vi "set_new_position.vi"(8 "error in (no error)":errorcluster, 10 "set_pos":dbl[](array[numeric]), 11 "dummyStage in":refnum<class "dummyStage.lvclass">) -> (0 "error out":errorcluster, 3 "dummyStage out":refnum<class "dummyStage.lvclass">)   [LabVIEW 2019, in "dummyStage.lvlib" / "dummyStage.lvclass"]
uses:
  dummyStage.lvclass
  subVIs/stage_idling.vi
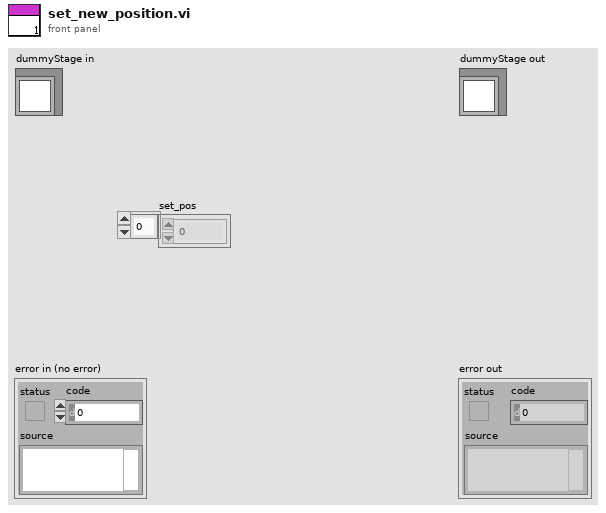
[diagram p1: front panel]
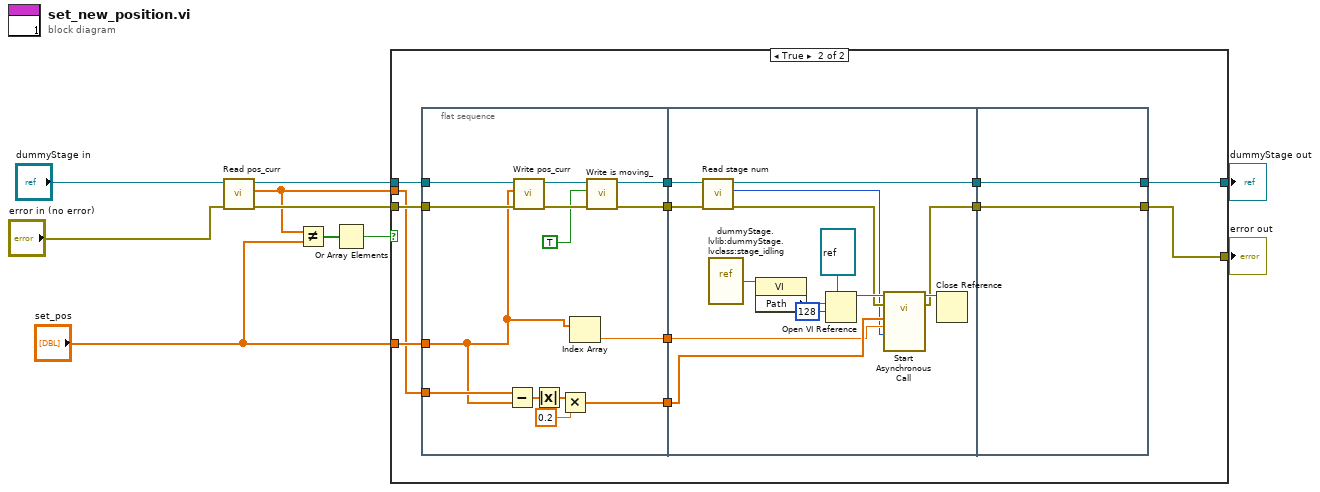
[diagram p0: block diagram]
diagram:
  n1 = call-dynamic "Read pos_curr.vi"("error in (no error)"="error in (no error)", "_stage in"="dummyStage in") -> ("error out"=w5:errorcluster, "readback position"=w4:dbl[], "_stage out"=w6:refnum<class "dummyStage.lvclass">)  [unwired: 7 in]
  n2 = Not Equal?(x=w4, y="set_pos") -> (x != y?=w2:bool[])
  n3 = Or Array Elements(Boolean array=w2) -> (logical OR=w1:bool)
  n4 = case shown="True" w1 {
    tunnel: [w12 w14] -> w9
    tunnel: [w11 w15] -> w7
    tunnel: w6 -> [w12 w24]
    tunnel: w5 -> [w11 w23]
    tunnel: w4 -> [_ w19]
    tunnel: "set_pos" -> [_ w22]
    frame False {
    }
    frame True {
      n5 = flat-sequence {
        tunnel: w22 -> [w26]
        tunnel: w23 -> [w32]
        tunnel: w24 -> [w33]
        tunnel: [w34] -> w21
        tunnel: [w30] -> w20
        tunnel: w19 -> [w35]
        tunnel: [w28] -> w18
        tunnel: [w25] -> w13
        tunnel: w21 -> [w48]
        tunnel: w20 -> [w43]
        tunnel: w18 -> [w41]
        tunnel: [w42] -> w17
        tunnel: [w45] -> w16
        tunnel: w13 -> [w47]
        tunnel: [w53] -> w15
        tunnel: [w54] -> w14
        tunnel: w17 -> [w54]
        tunnel: w16 -> [w53]
        frame #0 {
          n6 = Subtract(x=w35, y=w26) -> (x-y=w37:dbl[])
          n7 = call-dynamic "Write pos_curr.vi"("error in (no error)"=w32, "set_pos"=w26, "_stage in"=w33) -> ("error out"=w29:errorcluster, "_stage out"=w31:refnum<class "dummyStage.lvclass">)  [unwired: 7 in]
          n8 = Absolute Value(x=w37) -> (abs(x)=w38:dbl[])
          n9 = Multiply(x=w38, y=0.2) -> (x*y=w34:dbl[])
          n10 = Index Array(array=w26) -> (element=w25:dbl)  [unwired: 1 in]
          n11 = call-dynamic "Write is moving_.vi"("error in (no error)"=w29, "is moving?"=TRUE, "_stage in"=w31) -> ("error out"=w28:errorcluster, "_stage out"=w30:refnum<class "dummyStage.lvclass">)  [unwired: 7 in]
        }
        frame #1 {
          n12 = call-dynamic "Read stage num.vi"("error in (no error)"=w41, "_stage in"=w43) -> ("error out"=w40:errorcluster, "stage num"=w39:u8, "_stage out"=w42:refnum<class "dummyStage.lvclass">)  [unwired: 7 in]
          n13 = vi-ref "dummyStage.lvlib:dummyStage.lvclass:stage_idling.vi"() -> (w51:refnum<vi>)
          n14 = property class="VI"(reference=w51) -> ("Path"=w50:path)  [unwired: 1 in, 2 out]
          n15 = Open VI Reference(type specifier VI Refnum (for type only)=refnum<vi> refnum, vi path=w50, options=128) -> (vi reference=w49:refnum<vi>)  [unwired: 3 in, 1 out]
          n16 = call-by-ref "Start Asynchronous Call"(reference=w49, error in=w40, "num"=w39, "pos"=w47, "Array"=w48) -> (reference out=w46:refnum<vi>, error out=w45:errorcluster)  [unwired: 9 in]
          n17 = Close Reference(reference=w46) -> ()  [unwired: 1 in, 1 out]
        }
        frame #2 {
        }
      }
    }
  }
  "error out" <- w7
  "dummyStage out" <- w9
